vi "dotNET Parse Measurement Parameters.vi"(8 "error in":errorcluster) -> (0 "error out":errorcluster, 3 "Measurement Parameters":T1)   [LabVIEW 2020, in "Measurement Client Wrapper.lvclass"]
uses:
  Measurement Client Wrapper.lvclass
  Typedefs/Measurement Parameters.ctl
  Typedefs/Measurement Parameter Details.ctl
  Typedefs/Measurement DataType.ctl
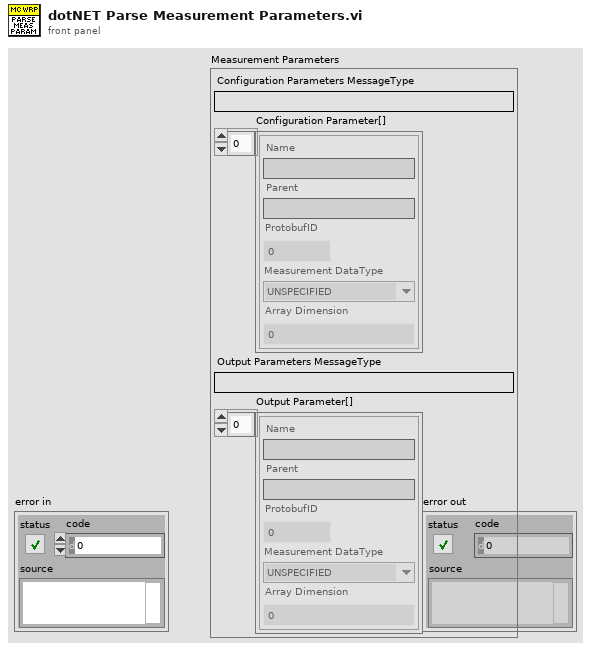
[diagram p1: front panel]
types:
  T1 = typedef "Measurement Client Wrapper.lvclass/Measurement Parameters.ctl" = cluster{"Configuration Parameters MessageType":string, "Configuration Parameter[]":T2[], "Output Parameters MessageType":string, "Output Parameter[]":T2[]}
  T2 = typedef "Measurement Client Wrapper.lvclass/Measurement Parameter Details.ctl" = cluster{"Name":string, "Parent":string, "ProtobufID":i32, "Measurement DataType":T3, "Array Dimension":i32}
  T3 = typedef "Measurement Client Wrapper.lvclass/Measurement DataType.ctl" = enum16{"UNSPECIFIED", "BOOL", "DOUBLE", "FLOAT", "INT32", "INT64", "STRING", "UINT32", "UINT64"}
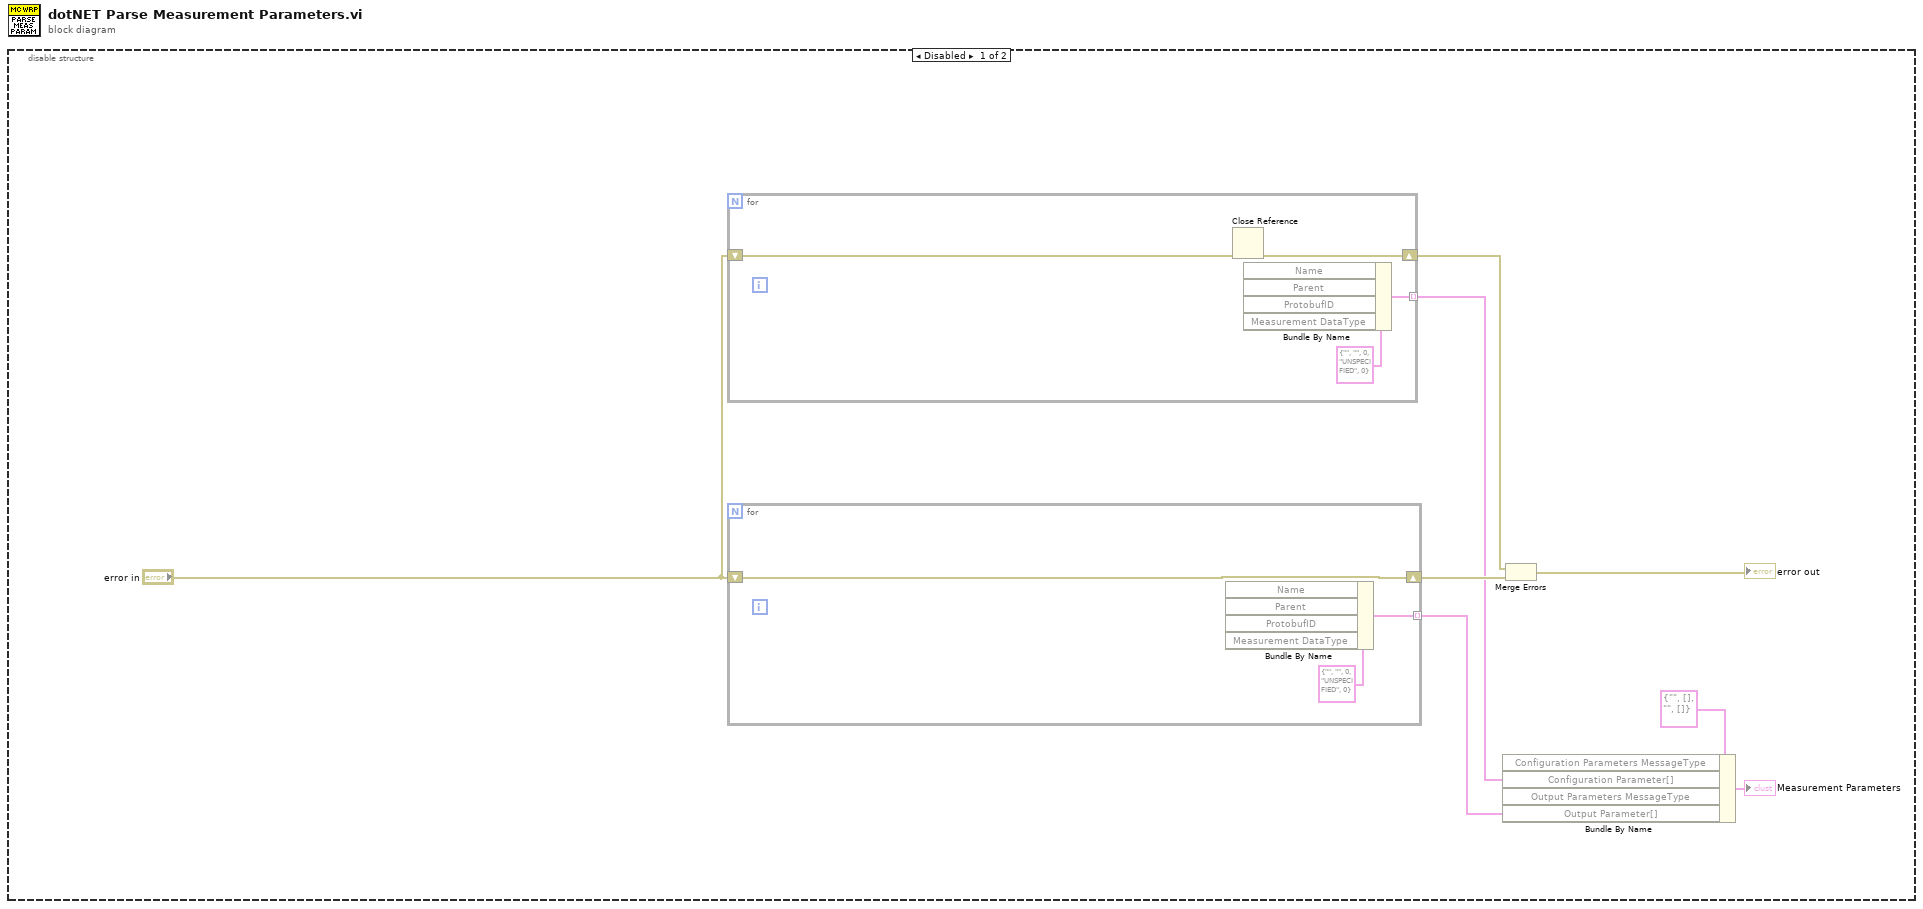
[diagram p0: block diagram]
diagram:
  n1 = disable-structure shown="Disabled" {
    frame Disabled {
      n2 = for {
        shift-right: [w14] -> w7
        shift-left: "error in" -> [w15]
        tunnel: [w12] -> w3 mode=indexing
        n3 = Close Reference(error in (no error)=w15) -> (error out=w14:errorcluster)  [unwired: 1 in]
        n4 = Bundle By Name(cluster=T2 {"Name"="", "Parent"="", "ProtobufID"=0, "Measurement DataType"=enum."UNSPECIFIED", "Array Dimension"=0} ("Measurement Parameter Details")) -> (w12:T2)  [unwired: 4 in]
      }
      n5 = for {
        shift-right: [w11] -> w6
        shift-left: "error in" -> [w11]
        tunnel: [w9] -> w2 mode=indexing
        n6 = Bundle By Name(cluster=T2 {"Name"="", "Parent"="", "ProtobufID"=0, "Measurement DataType"=enum."UNSPECIFIED", "Array Dimension"=0} ("Measurement Parameter Details")) -> (w9:T2)  [unwired: 4 in]
      }
      n7 = Bundle By Name(cluster=T1 {"Configuration Parameters MessageType"="", "Configuration Parameter[]"=[], "Output Parameters MessageType"="", "Output Parameter[]"=[]} ("Measurement Parameters"), "Configuration Parameter[]"=w3, "Output Parameter[]"=w2) -> (→"Measurement Parameters":T1)  [unwired: 2 in]
      n8 = Merge Errors(w7, w6) -> (→"error out":errorcluster)
    }
    frame Enabled {
    }
  }
